vi "updateUser.vi"(11 "Username":string) -> ()   [LabVIEW 2020, in "userLibrary.lvlib"]
uses:
  userLibrary.lvlib
  <vilib>/measure/mamon.llb/Trigger Detection for 1 Channel.vi
  <vilib>/addons/database/Connection.llb/DB Tools Open Connec (String).vi
  <vilib>/addons/database/NI_Database_API.lvlib
  databaseLibrary.lvlib
  maintenanceLibrary.lvlib
  <vilib>/measure/NI_MAPro.lvlib
panel:
  out "status 2":bool
  out "status 1":bool
  out "Log Max row":i32
  in  "Cancel":bool
  in  "OK":bool
  in  "Is Admin?":enum32{"Yes", "No"}(radio)
  in  "Full Name":string
  out "Username 2":string caption="Username"
  # "Update User"
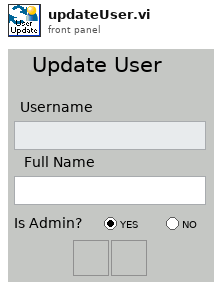
[diagram p1: front panel]
types:
  T1 = typedef "NI_Database_API.lvlib/Conn ObjectReference.ctl" = refnum<k1>
  T2 = cluster{"date/time string":string, "date/time string":string, "date/time string":string, string}
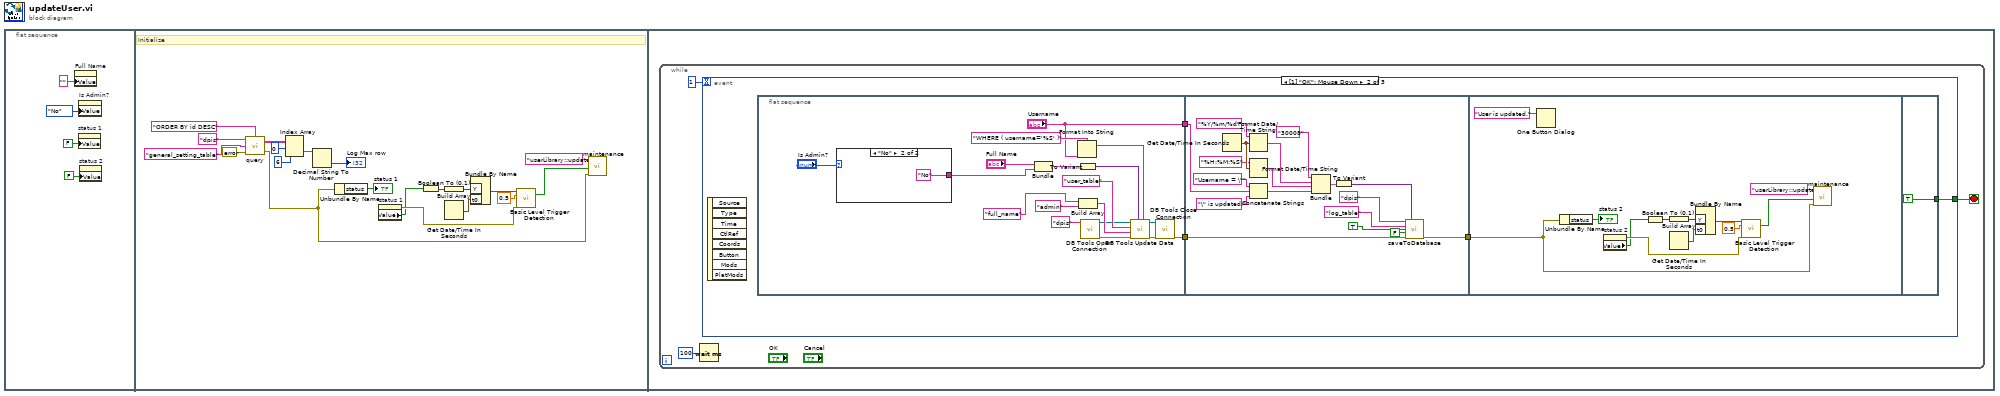
[diagram p0: block diagram]
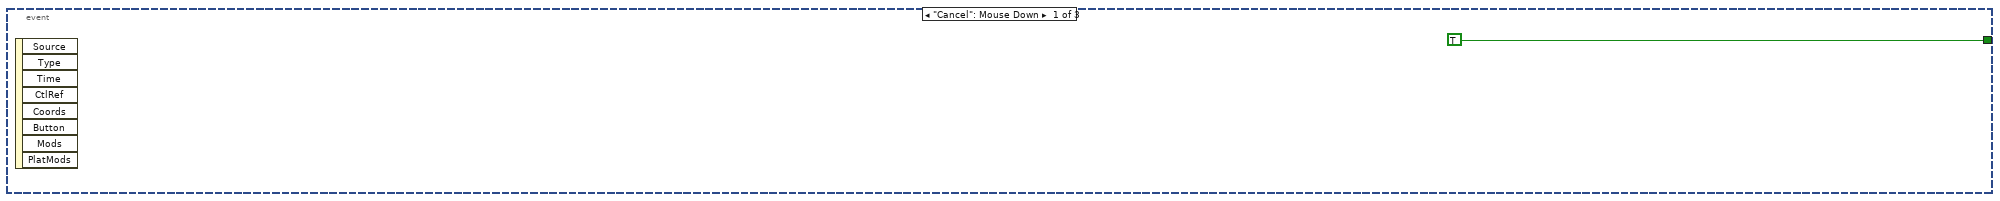
[diagram p2: hidden frame]
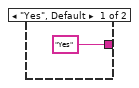
[diagram p3: hidden frame]
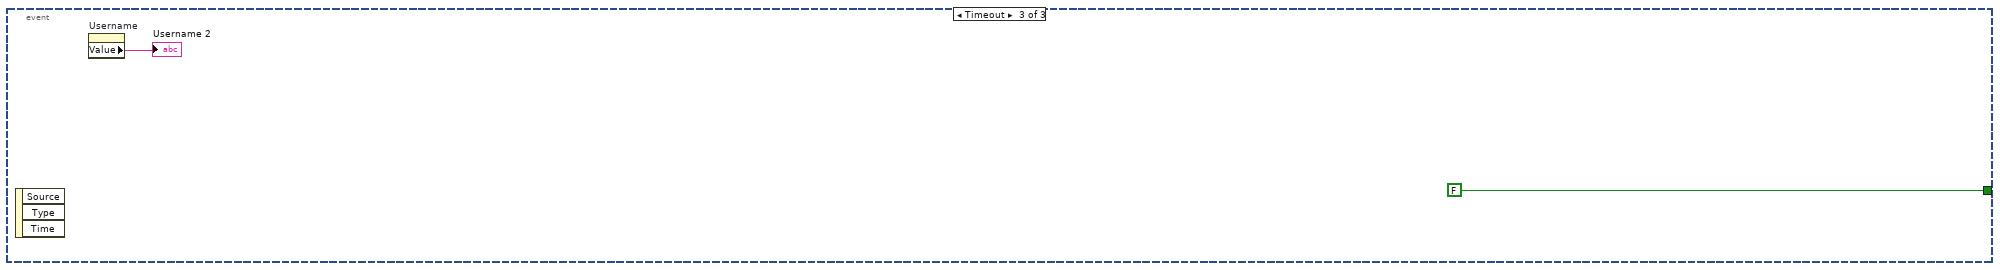
[diagram p4: hidden frame]
diagram:
  n1 = flat-sequence {
    frame #0 {
      n2 = property on="Full Name" class="Str"("Value"="" ("Full Name")) -> ()  [unwired: 2 in, 2 out]
      n3 = property on="status 1" class="Bool (strict)"("Value"=FALSE ("status 1")) -> ()  [unwired: 2 in, 2 out]
      n4 = property on="Is Admin?" class="RadioBtnsControl (strict)"("Value"=enum32{"Yes", "No"}."No" ("Is Admin?")) -> ()  [unwired: 2 in, 2 out]
      n5 = property on="status 2" class="Bool (strict)"("Value"=FALSE ("status 2")) -> ()  [unwired: 2 in, 2 out]
    }
    frame #1 {
      # "Initialize"
      n6 = call "query.vi"("Condition"="ORDER BY id DESC", "errorIn"=errorcluster {"status"=FALSE, "code"=0, "source"=""} ("Error in"), "Table Name"="general_setting_table", "Connection Name"="dpis") -> ("errorOut"=w5:errorcluster, "data"=w24:string[][])
      n7 = Index Array(array=w24, index (row)=0, index (col)=6 ("disabled index (col)")) -> (element=w17:string)
      n8 = Decimal String To Number(string=w17) -> (number=→"Log Max row":i32)  [unwired: 2 in, 1 out]
      n9 = Unbundle By Name(w5) -> ("status"=→"status 1":bool)
      n10 = property on="status 1" class="Bool (strict)"() -> (error out=w13:errorcluster, "Value"=w12:bool)  [unwired: 2 in, 1 out]
      n11 = Boolean To (0,1)(Boolean=w12) -> (0, 1=w8:i16)
      n12 = Build Array(w8) -> (w10:i16[])
      n13 = Get Date/Time In Seconds() -> (seconds since 1Jan1904=w9:timestamp)
      n14 = Bundle By Name("Y"=w10, "t0"=w9) -> (w11:waveform(i16))  [unwired: 1 in]
      n15 = call-poly <vilib>:"Basic Level Trigger Detection.vi"("signal in"=w11, "level"=0.5, "error in (no error)"=w13) -> ("trigger detected?"=w14:bool)  [unwired: 10 in, 2 out]
      n16 = call "maintenance.vi"("errorIn"=w5, "status"=w14, "errorLocation"="userLibrary::updateUser.vi::Initialize") -> ()  [unwired: 8 in, 1 out]
    }
    frame #2 {
      n17 = while {
        stop <- w27 stop-if-true
        n18 = Wait (ms)(milliseconds to wait=u32 100) -> ()  [unwired: 1 out]
        n19 = event shown="[1] \"OK\": Mouse Down" {
          selector: _ -> [_ _ _]
          dyn-events: _ -> [_ _ _]
          timeout: 1 -> [_ _ _]
          tunnel: [TRUE w31 FALSE] -> w27
          event "Cancel": Mouse Down {
            n20 = event-data() -> ()  [unwired: 1 in, 8 out]
          }
          event "OK": Mouse Down {
            n21 = event-data() -> ()  [unwired: 1 in, 8 out]
            n22 = flat-sequence {
              tunnel: [w36] -> w32
              tunnel: ["Username"] -> w30
              tunnel: w32 -> [w59]
              tunnel: w30 -> [w58]
              tunnel: [w56] -> w29
              tunnel: w29 -> [w71]
              tunnel: [TRUE] -> w31
              frame #0 {
                n23 = case shown="\"No\"" "Is Admin?" {
                  tunnel: ["Yes" ("table") "No" ("table")] -> w47
                  frame "Yes", Default {
                  }
                  frame "No" {
                  }
                }
                n24 = Bundle("Full Name"="Full Name", "table"=w47) -> (w38:cluster{"Full Name":string, "table":string})  [unwired: 1 in]
                n25 = Format Into String(format string="WHERE ( username='%S' )" ("condition"), "Username") -> (resulting string=w43:string)  [unwired: 2 in, 1 out]
                n26 = To Variant(anything=w38) -> (Variant=w37:variant)
                n27 = Build Array("full_name" ("table"), "admin" ("table")) -> (w41:string[])
                n28 = call-poly <vilib>:"DB Tools Open Connection.vi"("connection information"="dpis") -> ("error out"=w33:errorcluster, "connection reference"=w34:T1)  [unwired: 7 in]
                n29 = call <vilib>:"DB Tools Update Data.vi"("condition"=w43, "data"=w37, "error in (no error)"=w33, "columns"=w41, "table"="user_table", "connection reference"=w34) -> ("error out"=w45:errorcluster, "connection reference out"=w44:T1)  [unwired: 4 in]
                n30 = call <vilib>:"DB Tools Close Connection.vi"("error in (no error)"=w45, "connection reference"=w44) -> ("error out"=w36:errorcluster)  [unwired: 5 in]
              }
              frame #1 {
                n31 = Get Date/Time In Seconds() -> (seconds since 1Jan1904=w66:timestamp)
                n32 = Format Date/Time String(time format string (%c)="%Y/%m/%d", seconds (now)=w66) -> (date/time string=w67:string)  [unwired: 1 in]
                n33 = Format Date/Time String(time format string (%c)="%H:%M:%S", seconds (now)=w66) -> (date/time string=w68:string)  [unwired: 1 in]
                n34 = Concatenate Strings("Username = \"" ("string"), w58, "\" is updated." ("string")) -> (w65:string)
                n35 = Bundle("date/time string"="30008", "date/time string"=w67, "date/time string"=w68, w65) -> (w69:T2)  [unwired: 1 in]
                n36 = To Variant(anything=w69) -> (Variant=w70:variant)
                n37 = call "saveToDatabase.vi"("Connection"="dpis" ("table"), "Data"=w70, "Table"="log_table" ("table"), "Auto Increment ID?"=TRUE, "Delete row?"=FALSE, "Error in"=w59) -> ("Error out"=w56:errorcluster)  [unwired: 9 in]
              }
              frame #2 {
                n38 = One Button Dialog(message="User is updated.") -> ()  [unwired: 1 in, 1 out]
                n39 = Unbundle By Name(w71) -> ("status"=→"status 2":bool)
                n40 = property on="status 2" class="Bool (strict)"() -> (error out=w79:errorcluster, "Value"=w78:bool)  [unwired: 2 in, 1 out]
                n41 = Boolean To (0,1)(Boolean=w78) -> (0, 1=w74:i16)
                n42 = Build Array(w74) -> (w76:i16[])
                n43 = Get Date/Time In Seconds() -> (seconds since 1Jan1904=w75:timestamp)
                n44 = Bundle By Name("Y"=w76, "t0"=w75) -> (w77:waveform(i16))  [unwired: 1 in]
                n45 = call-poly <vilib>:"Basic Level Trigger Detection.vi"("signal in"=w77, "level"=0.5, "error in (no error)"=w79) -> ("trigger detected?"=w80:bool)  [unwired: 10 in, 2 out]
                n46 = call "maintenance.vi"("errorIn"=w71, "status"=w80, "errorLocation"="userLibrary::updateUser.vi::OK case") -> ()  [unwired: 8 in, 1 out]
              }
              frame #3 {
              }
            }
          }
          event Timeout {
            n47 = event-data() -> ()  [unwired: 1 in, 3 out]
            n48 = property on="Username" class="Str"() -> ("Value"=→"Username 2":string)  [unwired: 2 in, 2 out]
          }
        }
      }
    }
  }
